vi "PluginsLoaderService_Main.vi"(8 "error in (no error)":errorcluster, 9 "EventsOut":T1, 11 "PluginsLoaderService":refnum<class "PluginsLoaderService.lvclass">) -> ()   [LabVIEW 2014, in "PluginsThread.lvlib" / "PluginsLoaderService.lvclass"]
uses:
  PluginsLoaderService.lvclass
  _Plugins/_LVCMPlugin/GCMPlugin_EventsOut.ctl
  PluginsLoaderService_State.ctl
  _Plugins/GCMPlugin/GCMPlugin.lvclass
  PluginsLoaderService.lvclass/PluginsLoaderService.ctl
  _Plugins/_PluginLoader/_PluginLoader.lvclass
  ItemSelection/ItemSelection.lvlib
  PluginsLoaderCommander/PluginsLoaderCommander.lvclass
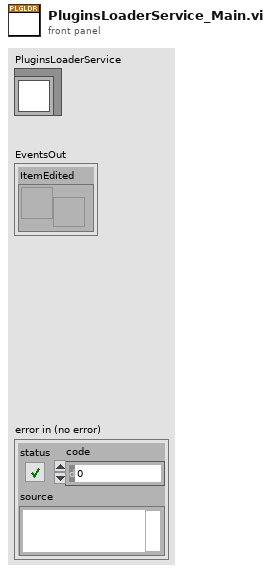
[diagram p1: front panel]
types:
  T1 = typedef "GCMPlugin.lvclass/GCMPlugin_EventsOut.ctl" = cluster{"ItemEdited":refnum<user-event>}
  T2 = typedef "PluginsThread.lvlib/PluginsLoaderService.lvclass/PluginsLoaderService_State.ctl" = enum16{"Initializing", "CheckingItemSelection", "CheckingCommands", "Stopping"}
  T3 = cluster{"CurrentItem":refnum<vi>, "AvailablePlugins":refnum<class "GCMPlugin.lvclass">[]}
  T4 = typedef "ItemSelection.lvlib/ItemSelection_Data.ctl" = cluster{"Command":T5, "Item Ref":T6}
  T5 = typedef "ItemSelection.lvlib/ItemSelection_Command.ctl" = enum16{"ItemSelected", "ItemUnselected"}
  T6 = typedef "ItemRef.ctl" = u64
  T7 = typedef "PluginsThread.lvlib/PluginsLoaderCommander.lvclass/PluginsLoaderCommander_Command.ctl" = enum16{"Stop", "Timeout"}
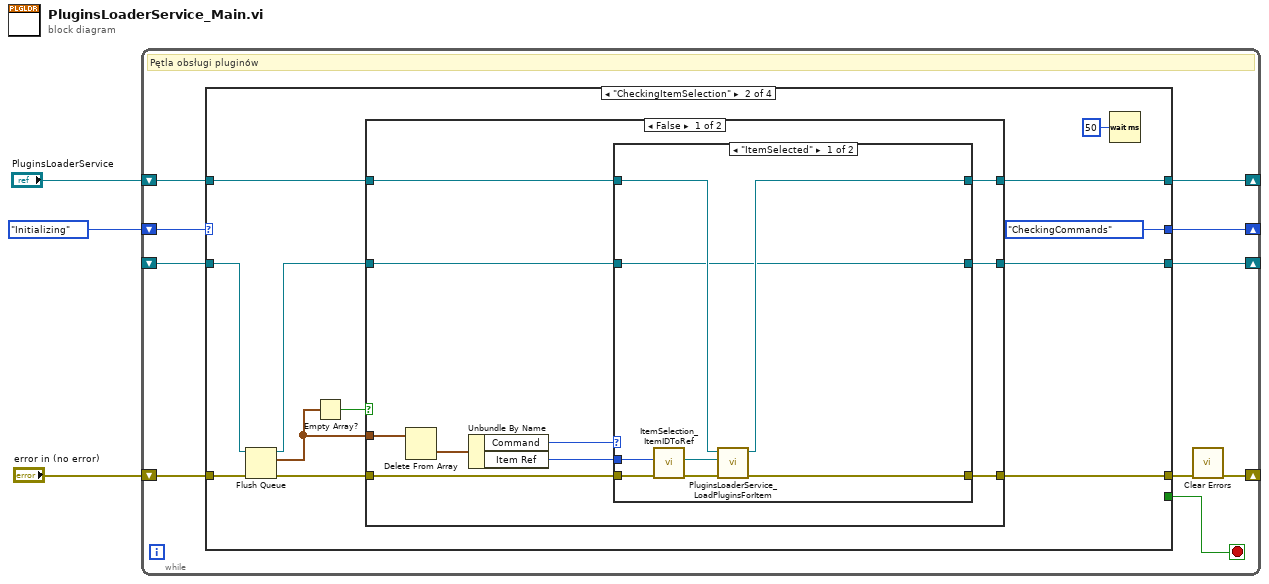
[diagram p0: block diagram]
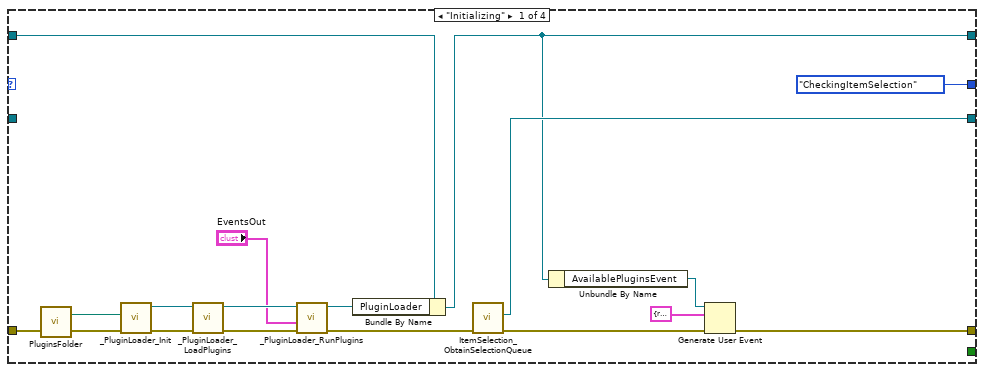
[diagram p2: hidden frame]
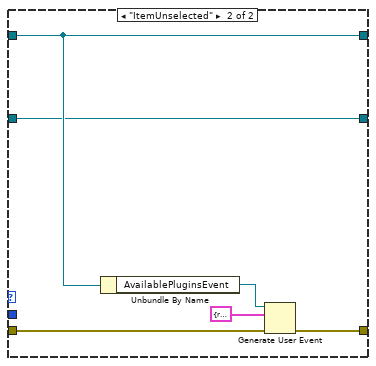
[diagram p3: hidden frame]
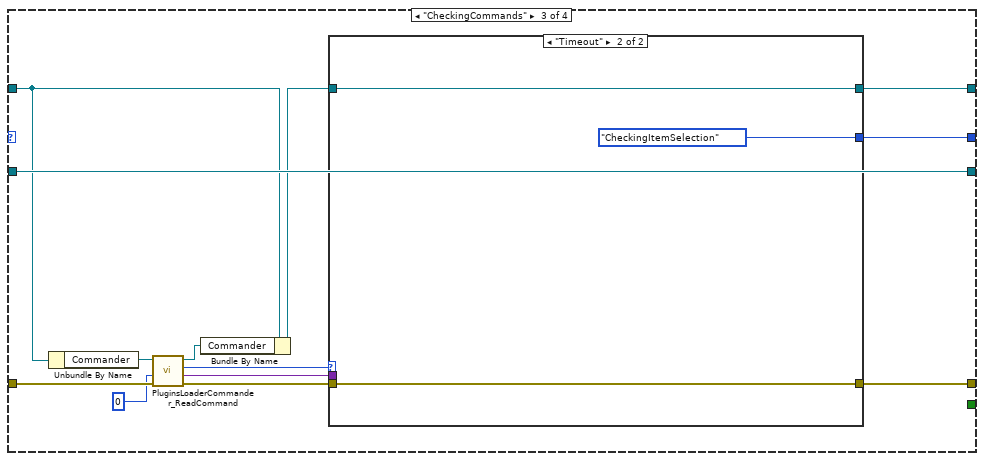
[diagram p5: hidden frame]
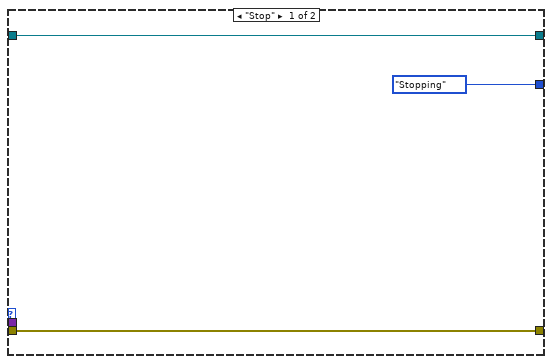
[diagram p6: hidden frame]
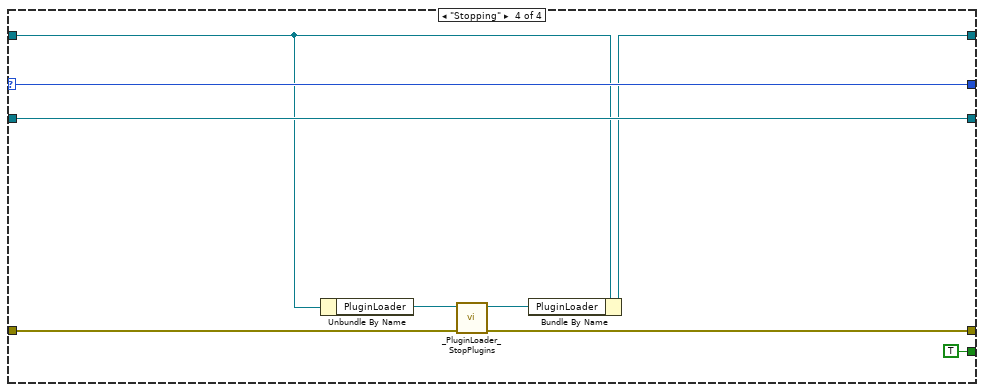
[diagram p7: hidden frame]
diagram:
  n1 = while {
    shift-right: [w8] -> _
    shift-left: PluginsLoaderService_State."Initializing" ("State") -> [w11]
    shift-right: [w7] -> _
    shift-left: "error in (no error)" -> [w12]
    shift-right: [w9] -> _
    shift-left: "PluginsLoaderService" -> [w10]
    shift-right: [w6] -> _
    shift-left: _ -> [w5]
    stop <- w4 stop-if-true
    # "Pętla obsługi pluginów"
    n2 = case shown="\"CheckingItemSelection\"" w11 {
      selector: w11 -> [_ _ _ w95]
      tunnel: [w14 w36 w75 w94] -> w13
      tunnel: w12 -> [w27 w42 w81 w89]
      tunnel: w10 -> [w26 w39 w78 w93]
      tunnel: [w15 w38 w77 w91] -> w9
      tunnel: [PluginsLoaderService_State."CheckingItemSelection" ("State") PluginsLoaderService_State."CheckingCommands" ("State") w70 w95] -> w8
      tunnel: [w19 w34 w82 w96] -> w6
      tunnel: w5 -> [_ w33 w82 w96]
      tunnel: [_ _ _ TRUE] -> w4
      frame "Initializing" {
        n3 = call "PluginsFolder.vi"() -> ("PluginsFolderPath"=w24:path)  [unwired: 3 in]
        n4 = call "_PluginLoader_Init.vi"("error in (no error)"=w27, "PluginsPath"=w24) -> ("error out"=w30:errorcluster, "_PluginLoader out"=w29:refnum<class "_PluginLoader.lvclass">)  [unwired: 8 in]
        n5 = call "_PluginLoader_LoadPlugins.vi"("error in (no error)"=w30, "_PluginLoader in"=w29) -> ("error out"=w28:errorcluster, "_PluginLoader out"=w23:refnum<class "_PluginLoader.lvclass">)  [unwired: 8 in]
        n6 = call "_PluginLoader_RunPlugins.vi"("error in (no error)"=w28, "EventsOut"="EventsOut", "_PluginLoader in"=w23) -> ("error out"=w20:errorcluster, "_PluginLoader out"=w22:refnum<class "_PluginLoader.lvclass">)  [unwired: 7 in]
        n7 = Bundle By Name(cluster=w26, "PluginLoader"=w22) -> (w15:refnum<class "PluginsLoaderService.lvclass">)
        n8 = call "ItemSelection_ObtainSelectionQueue.vi"("error in (no error)"=w20) -> ("error out"=w16:errorcluster, "queue out"=w19:refnum<queue>)  [unwired: 9 in]
        n9 = Unbundle By Name(w15) -> ("AvailablePluginsEvent"=w18:refnum<user-event>)
        n10 = Generate User Event(user event=w18, event data cluster=T3 {"CurrentItem"=refnum, "AvailablePlugins"=[]} ("event data"), error in=w16) -> (error out=w14:errorcluster)  [unwired: 1 in, 1 out]
      }
      frame "CheckingItemSelection" {
        n11 = Flush Queue(queue=w33, error in (no error)=w42) -> (queue out=w32:refnum<queue>, remaining elements=w40:T4[], error out=w35:errorcluster)
        n12 = Empty Array?(array=w40) -> (empty?=w37:bool)
        n13 = case shown="False" w37 {
          tunnel: w40 -> [w52 _]
          tunnel: w39 -> [w46 w68]
          tunnel: [w45 w68] -> w38
          tunnel: [w49 w69] -> w36
          tunnel: w35 -> [w48 w69]
          tunnel: w32 -> [w44 w67]
          tunnel: [w43 w67] -> w34
          frame False {
            n14 = Delete From Array(array=w52) -> (deleted portion=w51:T4)  [unwired: 2 in, 1 out]
            n15 = Unbundle By Name(w51) -> ("Command"=w50:T5, "Item Ref"=w47:T6)
            n16 = case shown="\"ItemSelected\"" w50 {
              tunnel: [w54 w64] -> w49
              tunnel: w48 -> [w59 w63]
              tunnel: w47 -> [w60 _]
              tunnel: w46 -> [w56 w62]
              tunnel: [w55 w62] -> w45
              tunnel: w44 -> [w53 w61]
              tunnel: [w53 w61] -> w43
              frame "ItemSelected" {
                n17 = call "ItemSelection_ItemIDToRef.vi"("error in (no error)"=w59, "Item"=w60) -> ("error out"=w58:errorcluster, "Item Refnum"=w57:refnum<vi>)  [unwired: 8 in]
                n18 = call "PluginsLoaderService_LoadPluginsForItem.vi"("error in (no error)"=w58, "ProjectItem"=w57, "PluginsLoaderService in"=w56) -> ("error out"=w54:errorcluster, "PluginsLoaderService out"=w55:refnum<class "PluginsLoaderService.lvclass">)  [unwired: 7 in]
              }
              frame "ItemUnselected" {
                n19 = Unbundle By Name(w62) -> ("AvailablePluginsEvent"=w66:refnum<user-event>)
                n20 = Generate User Event(user event=w66, event data cluster=T3 {"CurrentItem"=refnum, "AvailablePlugins"=[]} ("event data"), error in=w63) -> (error out=w64:errorcluster)  [unwired: 1 in, 1 out]
              }
            }
          }
          frame True {
          }
        }
        n21 = Wait (ms)(milliseconds to wait=u32 50) -> ()  [unwired: 1 out]
      }
      frame "CheckingCommands" {
        n22 = Unbundle By Name(w78) -> ("Commander"=w80:refnum<class "PluginsLoaderCommander.lvclass">)
        n23 = call "PluginsLoaderCommander_ReadCommand.vi"("error in (no error)"=w81, "timeout in ms (-1)"=0, "PluginsLoaderCommander in"=w80) -> ("error out"=w76:errorcluster, "Data"=w73:variant, "Command"=w74:T7, "PluginsLoaderCommander out"=w71:refnum<class "PluginsLoaderCommander.lvclass">)  [unwired: 5 in]
        n24 = Bundle By Name(cluster=w78, "Commander"=w71) -> (w72:refnum<class "PluginsLoaderService.lvclass">)
        n25 = case shown="\"Timeout\"" w74 {
          tunnel: w72 -> [w84 w88]
          tunnel: [w84 w88] -> w77
          tunnel: w76 -> [w85 w87]
          tunnel: [w85 w87] -> w75
          tunnel: w73 -> [_ _]
          tunnel: [PluginsLoaderService_State."Stopping" ("State") PluginsLoaderService_State."CheckingItemSelection" ("State")] -> w70
          frame "Stop" {
          }
          frame "Timeout" {
          }
        }
      }
      frame "Stopping" {
        n26 = Unbundle By Name(w93) -> ("PluginLoader"=w92:refnum<class "_PluginLoader.lvclass">)
        n27 = call "_PluginLoader_StopPlugins.vi"("error in (no error)"=w89, "_PluginLoader in"=w92) -> ("error out"=w94:errorcluster, "_PluginLoader out"=w90:refnum<class "_PluginLoader.lvclass">)  [unwired: 8 in]
        n28 = Bundle By Name(cluster=w93, "PluginLoader"=w90) -> (w91:refnum<class "PluginsLoaderService.lvclass">)
      }
    }
    n29 = call <vilib>:"Clear Errors.vi"("error in (no error)"=w13) -> ("error out"=w7:errorcluster)  [unwired: 5 in, 1 out]
  }
